vi "read_tag_calibration.vi"(5 "tag_name":string, 7 "runtime":variant, 8 "error in (no error)":errorcluster) -> (0 "error out":errorcluster, 3 "calibration":T1={"tag_name"="", "type"="<type>", "offset"=0.0, "slope"=0.0, "formula"="", "x_points"=[], "y_points"=[]})   [LabVIEW 2015, in "lv-calibration.lvlib"]
uses:
  lv-calibration.lvlib
  _controls/runtime.ctl
  _controls/type.ctl
  _controls/error.ctl
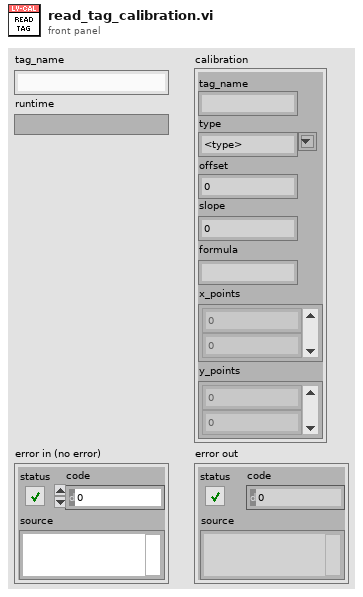
[diagram p1: front panel]
types:
  T1 = typedef "lv-calibration.lvlib/runtime.ctl" = cluster{"tag_name":string, "type":T2, "offset":dbl, "slope":dbl, "formula":string, "x_points":dbl[], "y_points":dbl[]}
  T2 = typedef "lv-calibration.lvlib/type.ctl" = string
  T3 = typedef "lv-calibration.lvlib/error.ctl" = enum16{"<error>", "unsupported_calibration_type", "tag_name_not_found", "duplicate_tag_names", "formula_empty"}
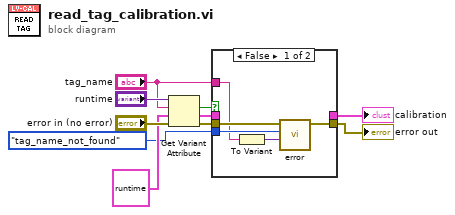
[diagram p0: block diagram]
diagram:
  n1 = Get Variant Attribute(Variant="runtime", name="tag_name", default value (empty Variant)=T1 {"tag_name"="", "type"="<type>", "offset"=0.0, "slope"=0.0, "formula"="", "x_points"=[], "y_points"=[]} ("calibration"), error in="error in (no error)") -> (found=w4:bool, value=w2:T1, error out=w5:errorcluster)  [unwired: 1 out]
  n2 = case shown="False" w4 {
    tunnel: [w15 w17] -> w7
    tunnel: error."tag_name_not_found" ("error") -> [w14 _]
    tunnel: w5 -> [w13 w17]
    tunnel: "tag_name" -> [w12 _]
    tunnel: w2 -> [_ w16]
    tunnel: [_ w16] -> w1
    frame False {
      n3 = To Variant(anything=w12) -> (Variant=w11:variant)
      n4 = call "error.vi"("data"=w11, "error"=w14, "error in (no error)"=w13) -> ("error out"=w15:errorcluster)  [unwired: 8 in]
    }
    frame True {
    }
  }
  "error out" <- w7
  "calibration" <- w1
